vi "testing nidaq device readback.vi"() -> ()   [LabVIEW 2021]
uses:
  <vilib>/DAQmx/read.llb/DAQmx Read (Digital 1D Bool NChan 1Samp 1Line).vi
  <vilib>/DAQmx/write.llb/DAQmx Write (Digital 1D Bool NChan 1Samp 1Line).vi
  <extravilib>/ChannelInstances/Tag-bool/Write With Abort.vi
  <extravilib>/ChannelInstances/Tag-bool/Read With Abort.vi
  <extravilib>/ChannelInstances/Tag-bool/Instantiate.vi
  <extravilib>/ChannelInstances/Tag-bool/Endpoint.vi
  <vilib>/DAQmx/miscellaneous.llb/DAQmx Fill In Error Info.vi
  <extravilib>/ChannelInstances/Tag-bool/EndpointRead.vi
  <extravilib>/ChannelInstances/Tag-bool.lvlib
panel:
  in  "Num Channels":i32=8
  in  "start button":bool
  in  "DAQmx Task Name":refnum<k21>
  out "async read cycle":i32
  out "async digital readback":bool[](array[boolean])
  out "sync. digital readback":bool[](array[boolean])
  out "write cycle":i32
  out "written digital output":bool[](array[boolean])
  in  "Stop":bool
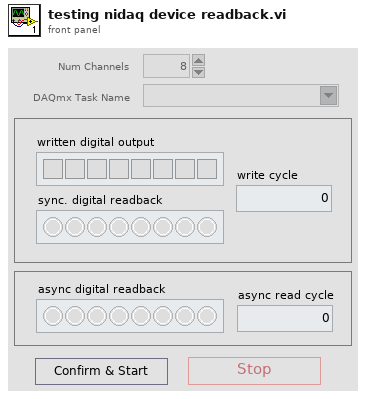
[diagram p1: front panel]
types:
  T1 = enum8{"Enabled", "Disabled", "Disabled and Grayed Out"}
  T2 = typedef "Tag-bool.lvlib/))Channel.ctl" = refnum<queue>
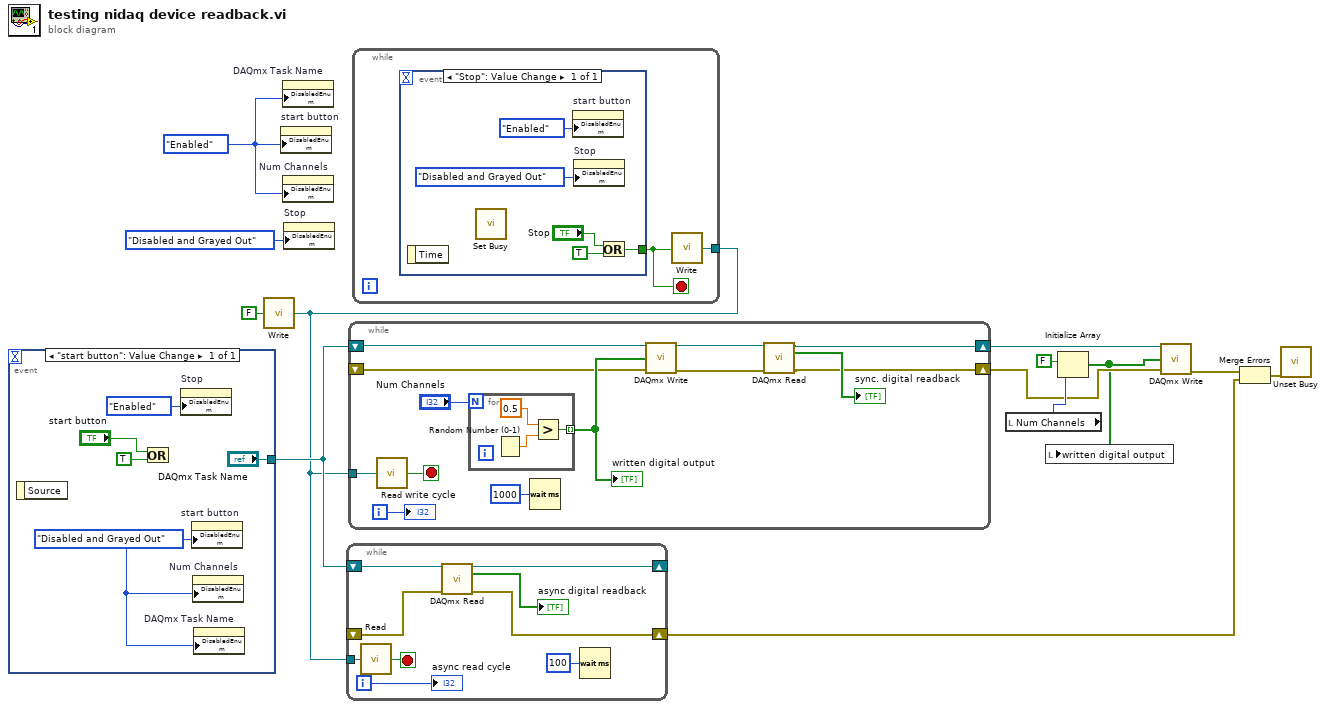
[diagram p0: block diagram]
diagram:
  w6 = T1."Enabled" ("Disabled")
  n1 = event shown="[0] \"start button\": Value Change" {
    selector: _ -> [_]
    dyn-events: _ -> [_]
    timeout: _ -> [_]
    tunnel: ["DAQmx Task Name"] -> w11
    event "start button": Value Change {
      w14 = T1."Disabled and Grayed Out" ("Disabled")
      n2 = event-data() -> ()  [unwired: 1 in, 1 out]
      n3 = Or(x="start button", y=TRUE) -> ()  [unwired: 1 out]
      n4 = property on="Stop" class="Bool"("DisabledEnum"=T1."Enabled" ("Disabled")) -> ()  [unwired: 2 in, 2 out]
      n5 = property on="start button" class="Bool"("DisabledEnum"=w14) -> ()  [unwired: 2 in, 2 out]
      n6 = property on="Num Channels" class="DigNum (strict)"("DisabledEnum"=w14) -> ()  [unwired: 2 in, 2 out]
      n7 = property on="DAQmx Task Name" class="DAQmxName (strict)"("DisabledEnum"=w14) -> ()  [unwired: 2 in, 2 out]
    }
  }
  n8 = call <extravilib>:"Write.vi"("element"=FALSE) -> ("channel"=w10:T2)  [unwired: 1 out]
  n9 = property on="start button" class="Bool"("DisabledEnum"=w6) -> ()  [unwired: 2 in, 2 out]
  n10 = property on="DAQmx Task Name" class="DAQmxName (strict)"("DisabledEnum"=w6) -> ()  [unwired: 2 in, 2 out]
  n11 = property on="Num Channels" class="DigNum (strict)"("DisabledEnum"=w6) -> ()  [unwired: 2 in, 2 out]
  n12 = property on="Stop" class="Bool"("DisabledEnum"=T1."Disabled and Grayed Out" ("Disabled")) -> ()  [unwired: 2 in, 2 out]
  n13 = while {
    tunnel: w10 -> [w26]
    shift-right: [w23] -> _
    shift-left: w11 -> [w24]
    shift-right: [w20] -> w2
    shift-left: _ -> [w19]
    i -> [w22]
    stop <- w27 stop-if-true
    n14 = call <extravilib>:"Read.vi"("channel"=w26) -> ("element"=w27:bool)  [unwired: 1 in, 1 out]
    n15 = call-poly <vilib>:"DAQmx Read.vi"("task/channels in"=w24, "error in"=w19) -> ("task out"=w23:refnum<k21>, "data"=→"async digital readback":bool[], "error out"=w20:errorcluster)  [unwired: 11 in]
    n16 = Wait (ms)(milliseconds to wait=u32 100) -> ()  [unwired: 1 out]
    "async read cycle" <- w22
  }
  n17 = while {
    tunnel: w10 -> [w37]
    shift-right: [w33] -> w9
    shift-left: w11 -> [w36]
    shift-right: [w29] -> w5
    shift-left: _ -> [w28]
    i -> [w38]
    stop <- w39 stop-if-true
    n18 = call <extravilib>:"Read.vi"("channel"=w37) -> ("element"=w39:bool)  [unwired: 1 in, 1 out]
    n19 = for {
      N: "Num Channels" -> [_]
      tunnel: [w41] -> w35 mode=indexing
      n20 = Random Number (0-1)() -> (number: 0 to 1=w43:dbl)
      n21 = Greater?(x=0.5, y=w43) -> (0:w41:bool)
    }
    "written digital output" <- w35
    n22 = Wait (ms)(milliseconds to wait=u32 1000) -> ()  [unwired: 1 out]
    n23 = call-poly <vilib>:"DAQmx Write.vi"("task/channels in"=w36, "data"=w35, "error in"=w28) -> ("task out"=w34:refnum<k21>, "error out"=w30:errorcluster)  [unwired: 10 in, 1 out]
    n24 = call-poly <vilib>:"DAQmx Read.vi"("task/channels in"=w34, "error in"=w30) -> ("task out"=w33:refnum<k21>, "data"=→"sync. digital readback":bool[], "error out"=w29:errorcluster)  [unwired: 11 in]
    "write cycle" <- w38
  }
  n25 = while {
    tunnel: w10 -> [w44]
    stop <- w45 stop-if-true
    n26 = event shown="[0] \"Stop\": Value Change" {
      selector: _ -> [_]
      dyn-events: _ -> [_]
      timeout: _ -> [_]
      tunnel: [w49] -> w45
      event "Stop": Value Change {
        n27 = event-data() -> ()  [unwired: 1 in, 1 out]
        n28 = call <vilib>:"Set Busy.vi"() -> ()  [unwired: 10 in, 2 out]
        n29 = property on="start button" class="Bool"("DisabledEnum"=T1."Enabled" ("Disabled")) -> ()  [unwired: 2 in, 2 out]
        n30 = property on="Stop" class="Bool"("DisabledEnum"=T1."Disabled and Grayed Out" ("Disabled")) -> ()  [unwired: 2 in, 2 out]
        n31 = Or(x="Stop", y=TRUE) -> (x .or. y?=w49:bool)
      }
    }
    n32 = call <extravilib>:"Write.vi"("element"=w45) -> ("channel"=w44:T2)  [unwired: 1 out]
  }
  n33 = local read "Num Channels"() -> (w7:i32)
  n34 = Initialize Array(FALSE, w7) -> (w1:bool[])
  n35 = local write "written digital output"(w1) -> ()
  n36 = call-poly <vilib>:"DAQmx Write.vi"("task/channels in"=w9, "data"=w1, "error in"=w5) -> ("error out"=w3:errorcluster)  [unwired: 10 in, 2 out]
  n37 = Merge Errors(w3, w2) -> (w4:errorcluster)
  n38 = call <vilib>:"Unset Busy.vi"("error in (no error)"=w4) -> ()  [unwired: 10 in, 1 out]
